vi "FR generate zmag.vi"(7 "exp fit":cluster{"A":dbl, "B":dbl}={"A"=28.47, "B"=-1.501}, 9 "每步加载率":dbl, 10 "终点":dbl, 11 "起点":dbl) -> (0 "Wrong":bool, 2 "FR zmag":dbl[](array[numeric]))   [LabVIEW 2017]
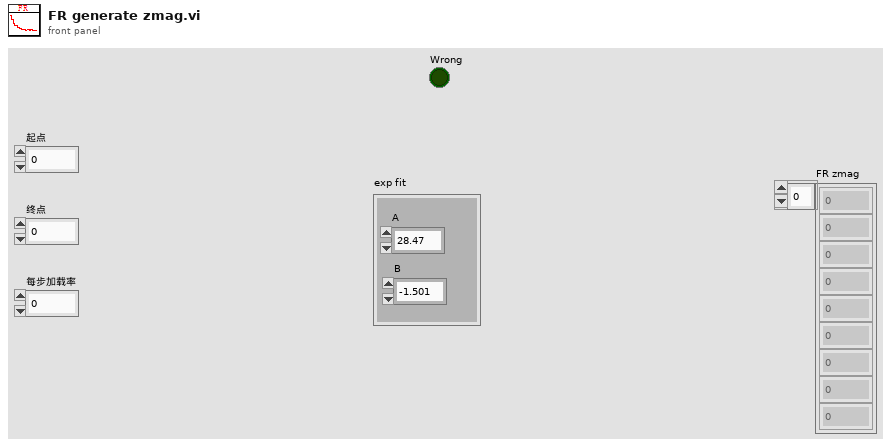
[diagram p1: front panel]
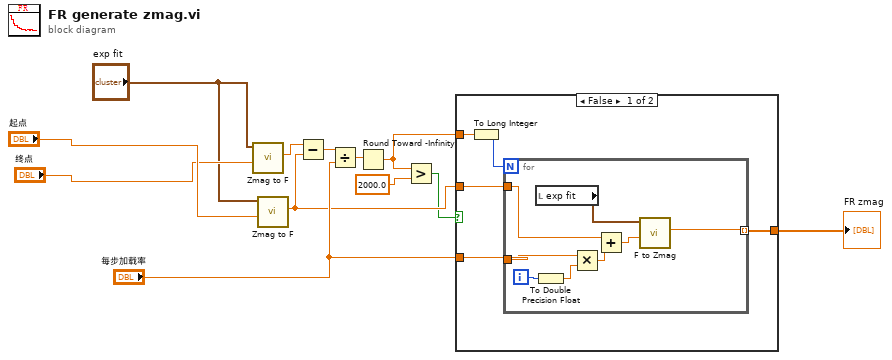
[diagram p0: block diagram]
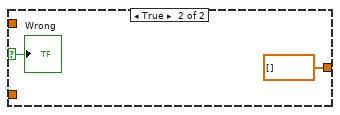
[diagram p2: hidden frame]
diagram:
  n1 = call "Zmag to F.vi"("Z 输入"="终点", "Parameter T1"="exp fit") -> ("F 输出"=w7:dbl)  [unwired: 9 in]
  n2 = call "Zmag to F.vi"("Z 输入"="起点", "Parameter T1"="exp fit") -> ("F 输出"=w6:dbl)  [unwired: 9 in]
  n3 = Subtract(x=w7, y=w6) -> (x-y=w5:dbl)
  n4 = Divide(x=w5, y="每步加载率") -> (x/y=w4:dbl)
  n5 = Round Toward -Infinity(1:w4) -> (0:w3:dbl)
  n6 = Greater?(x=w3, y=2000.0) -> (0:w1:bool)
  n7 = case shown="False" w1 {
    selector: w1 -> [_ w26]
    tunnel: w6 -> [w17 _]
    tunnel: "每步加载率" -> [w15 _]
    tunnel: [w14 dbl[] []] -> w10
    tunnel: w3 -> [w13 _]
    frame False {
      n8 = To Long Integer(number=w13) -> (32bit integer=w16:i32)
      n9 = for {
        N: w16 -> [_]
        tunnel: w17 -> [w21]
        tunnel: w15 -> [w24]
        tunnel: [w19] -> w14 mode=indexing
        i -> [w25]
        n10 = local read "exp fit"() -> (w18:cluster{"A":dbl, "B":dbl})
        n11 = To Double Precision Float(number=w25) -> (double precision float=w23:dbl)
        n12 = Multiply(x=w24, y=w23) -> (x*y=w22:dbl)
        n13 = Add(x=w21, y=w22) -> (x+y=w20:dbl)
        n14 = call "F to Zmag.vi"("F输入"=w20, "Parameter T1"=w18) -> ("Z输出"=w19:dbl)  [unwired: 9 in]
      }
    }
    frame True {
      "Wrong" <- w26
    }
  }
  "FR zmag" <- w10
